vi "Main Engine.vi"() -> ()   [LabVIEW 2014, in "Dragon Tamers.lvlib"]
uses:
  Dragon Tamers.lvlib
  Typedefs/Queue Commands.ctl
  Typedefs/Main Cluster.ctl
  Typedefs/Config File Cluster.ctl
  Typedefs/Paths.ctl
  Typedefs/Input Parsed.ctl
  Typedefs/King.ctl
  Typedefs/Cell Pos.ctl
  Typedefs/Board.ctl
  Typedefs/Board Cell.ctl
  Typedefs/Cell Occupancy.ctl
  <vilib>/Utility/config.llb/NI_LVConfig.lvlib
  <vilib>/Utility/error.llb/DialogType.ctl
panel:
  out "Debug Board 2D String":string[][](table)
  out "Output Text":string
  out "Total Plays":i32=1
  out "Our Team":i32
  in  "Continue?":bool
  in  "Next Button":bool
  in  "Play Number":i32=1
  in  "Debug?":bool
  in  "Stop Waiting":bool
  out "Status":string
  in  "Stop Button":bool
  # "Dragon Tamers!"
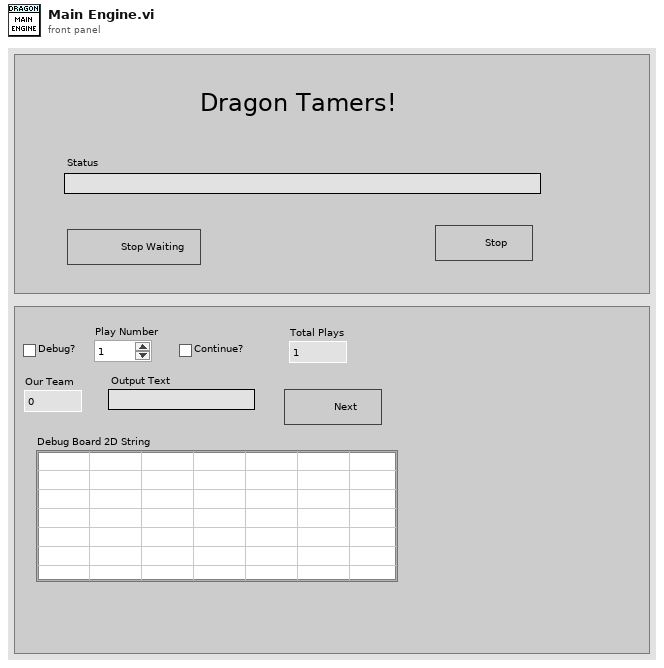
[diagram p1: front panel]
types:
  T1 = typedef "Dragon Tamers.lvlib/Queue Commands.ctl" = enum16{"Create", "Enqueue", "Enqueue N", "Enstack", "Dequeue", "Flush", "Release"}
  T2 = typedef "Dragon Tamers.lvlib/Main Cluster.ctl" = cluster{string, "Config":T3, "Paths":T4, "Play Number":i32, "Input Parsed":T5, "Output Text":string, "File List to Monitor":string[]}
  T3 = typedef "Dragon Tamers.lvlib/Config File Cluster.ctl" = cluster{"File Directory":path}
  T4 = typedef "Dragon Tamers.lvlib/Paths.ctl" = cluster{"App Directory":path, "Config File":path}
  T5 = typedef "Dragon Tamers.lvlib/Input Parsed.ctl" = cluster{"Our Team":i32, "King":T6, "Board":T8, "1D Board":T9[]}
  T6 = typedef "Dragon Tamers.lvlib/King.ctl" = cluster{"Set King?":bool, "Min":i32, "Max":i32, "DT Swap Count":i32, "Opp. Swap Count":i32, "DT Pos.":T7, "Opp. Pos.":T7}
  T7 = typedef "Dragon Tamers.lvlib/Cell Pos.ctl" = cluster{"X":i32, "Y":i32}
  T8 = typedef "Dragon Tamers.lvlib/Board.ctl" = T9[][]
  T9 = typedef "Dragon Tamers.lvlib/Board Cell.ctl" = cluster{"Team":i32, "Occu.":T10, "Count":i32}
  T10 = typedef "Dragon Tamers.lvlib/Cell Occupancy.ctl" = enum16{"N", "C", "K"}
  T11 = typedef "Dragon Tamers.lvlib/Parsed Board.ctl" = cluster{"DT King":i32, "Opp King":i32, "Count":i32[], "Empty Cells":i32[], "DT Cells":i32[], "Opp Cells":i32[], "DT Team":i32, "Opp. Team":i32}
  T12 = typedef "NI_LVConfig.lvlib/Config Data RefNum.ctl" = refnum<k1>
  T13 = typedef "DialogType.ctl" = u16
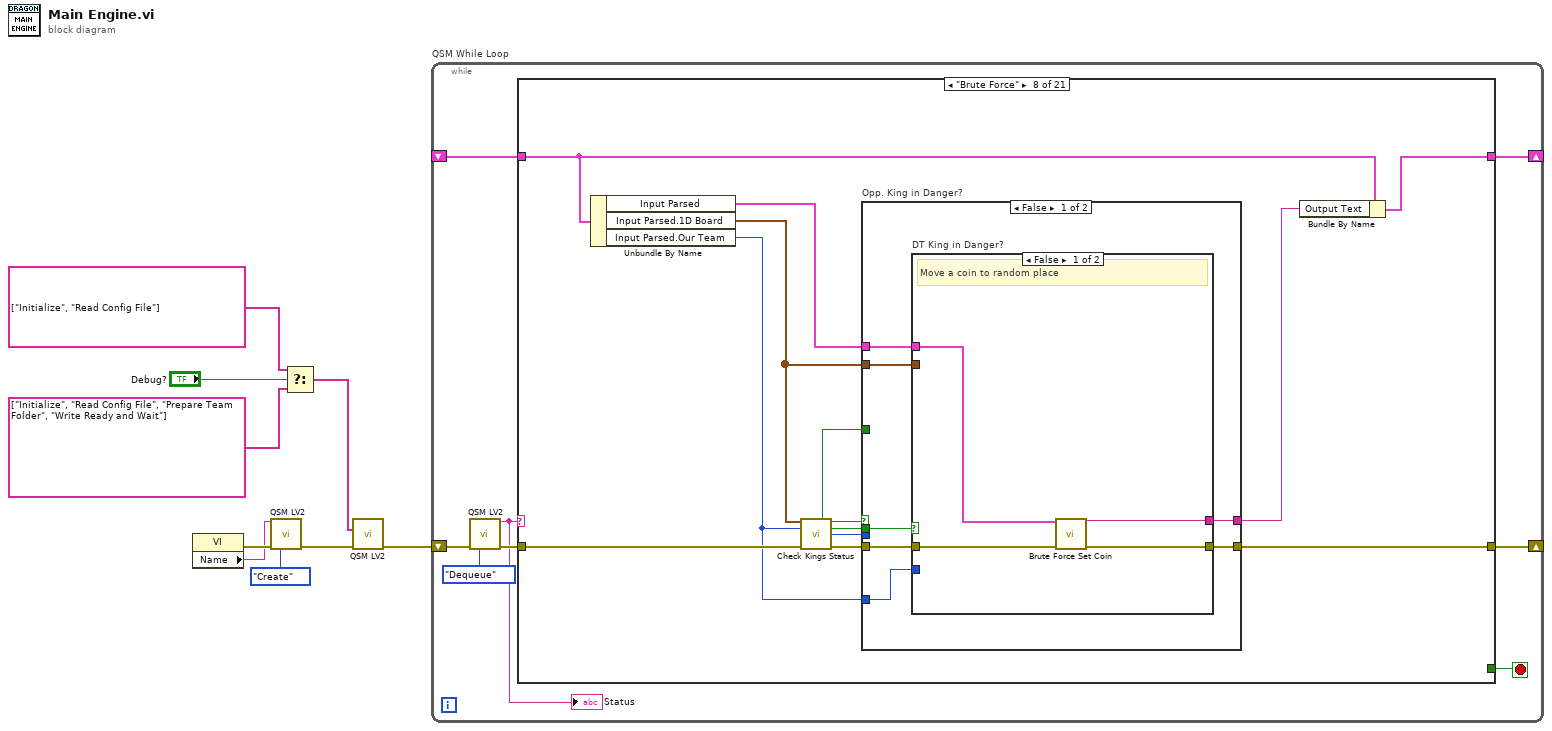
[diagram p0: block diagram]
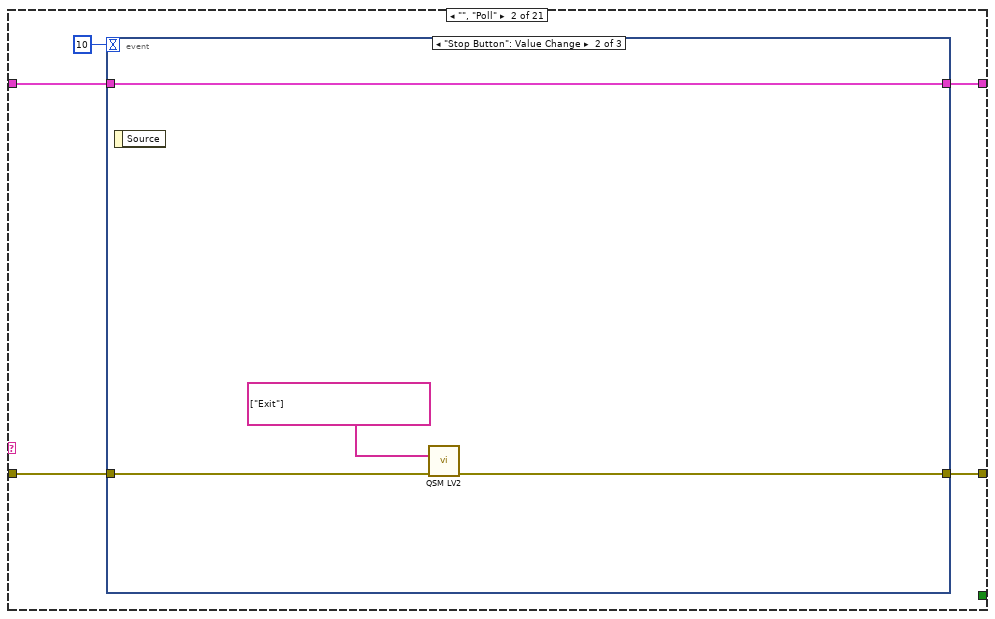
[diagram p3: hidden frame]
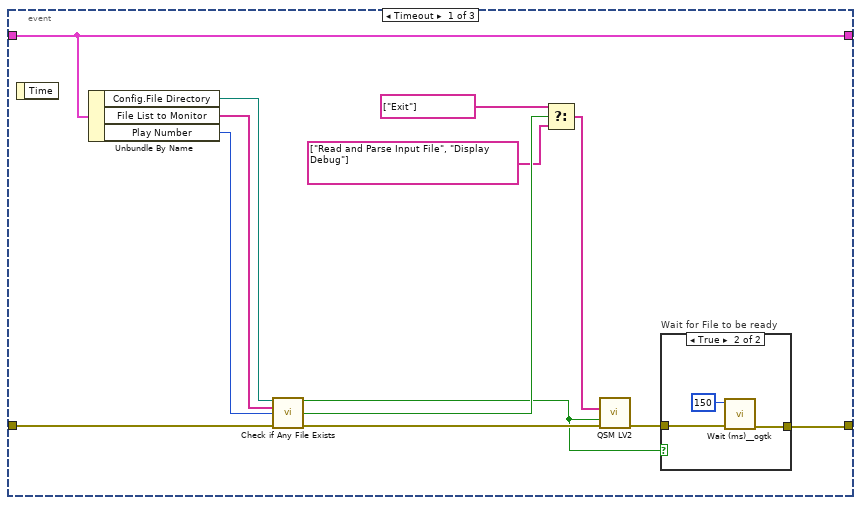
[diagram p4: hidden frame]
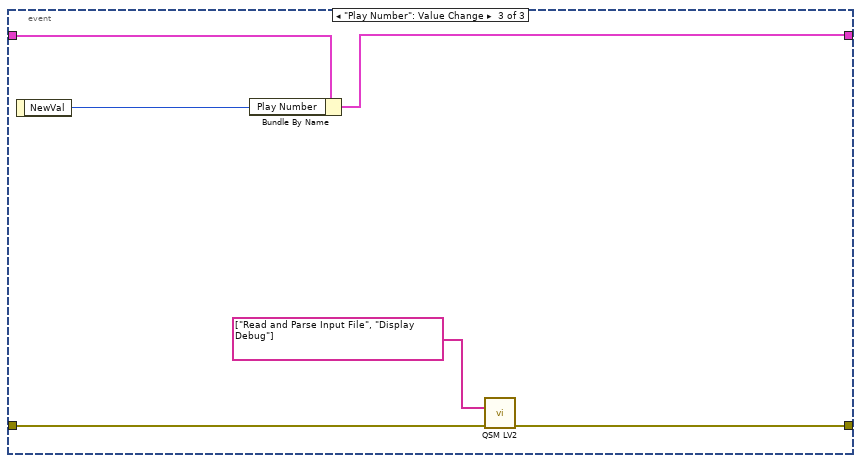
[diagram p6: hidden frame]
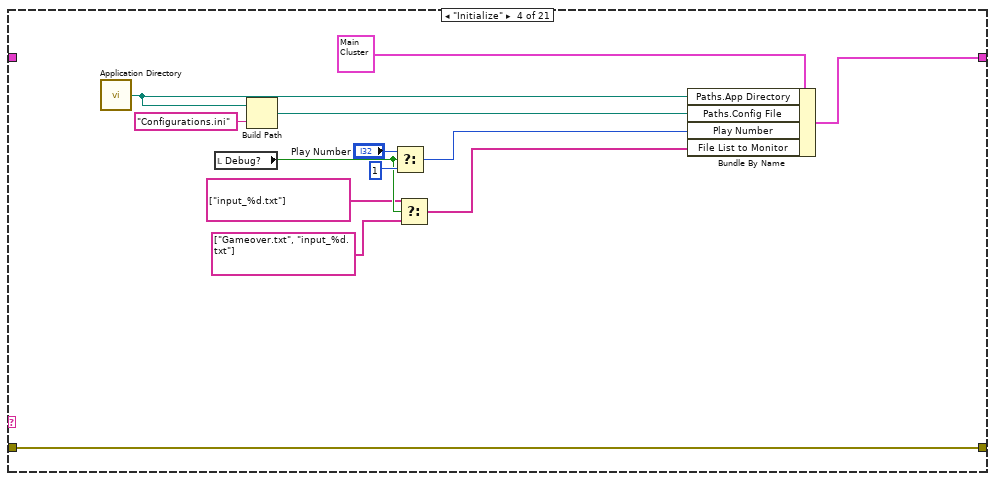
[diagram p8: hidden frame]
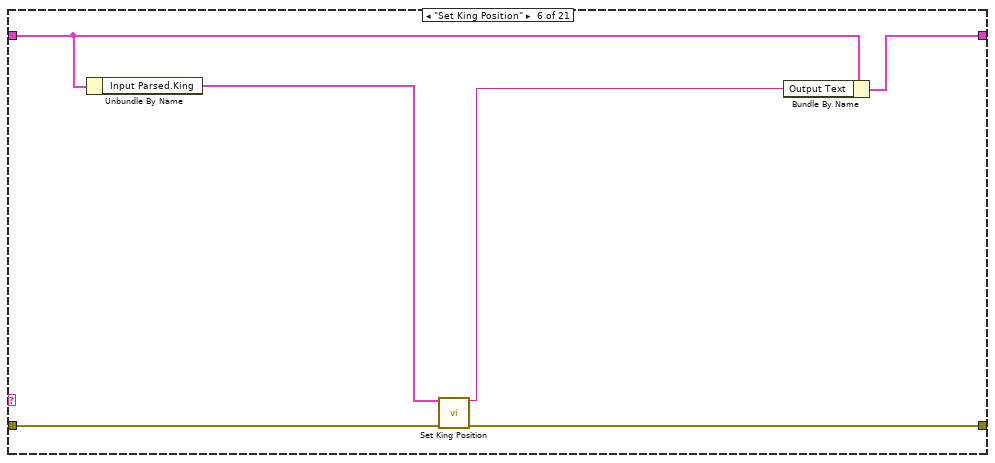
[diagram p10: hidden frame]
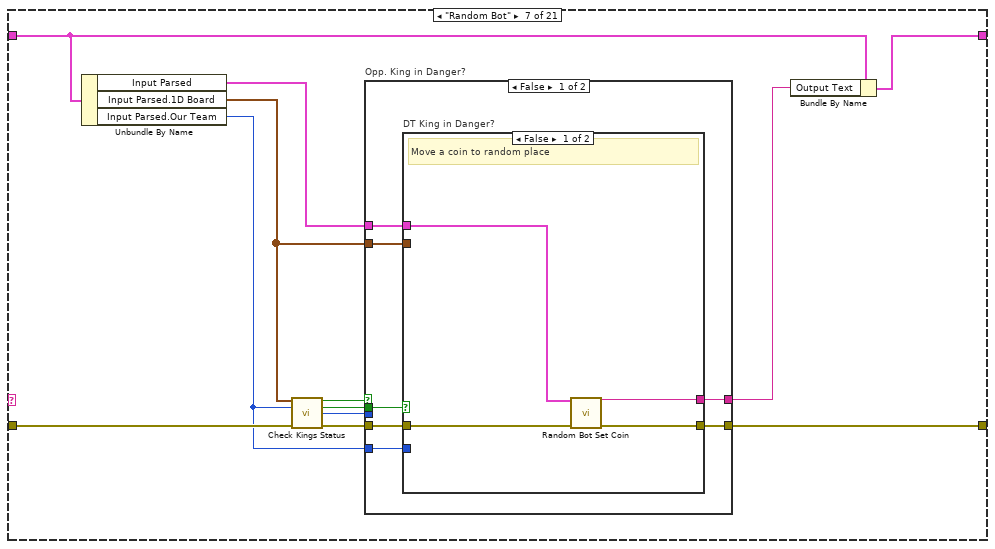
[diagram p11: hidden frame]
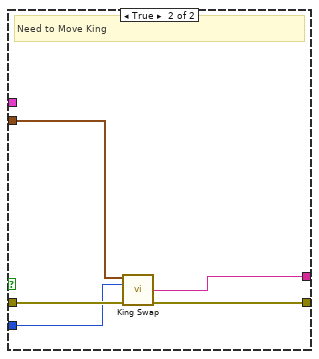
[diagram p12: hidden frame]
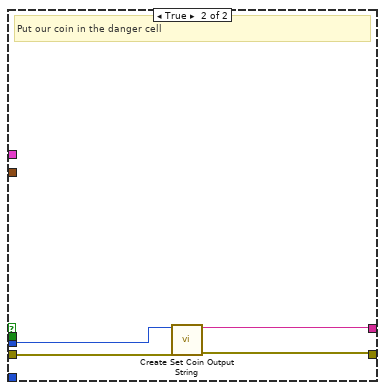
[diagram p13: hidden frame]
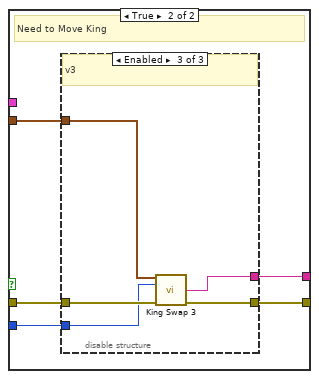
[diagram p14: hidden frame]
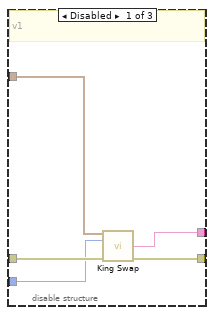
[diagram p15: hidden frame]
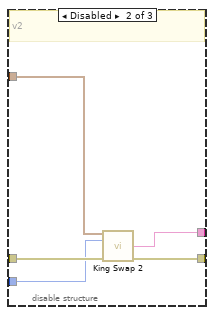
[diagram p16: hidden frame]
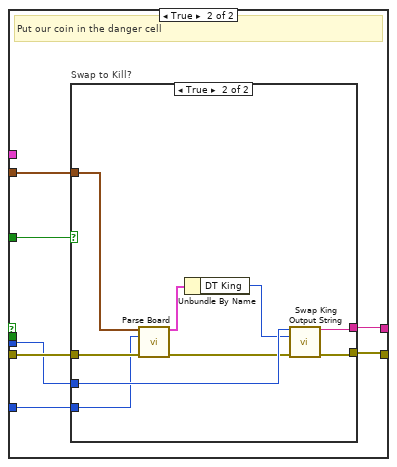
[diagram p17: hidden frame]
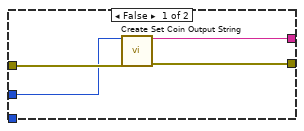
[diagram p18: hidden frame]
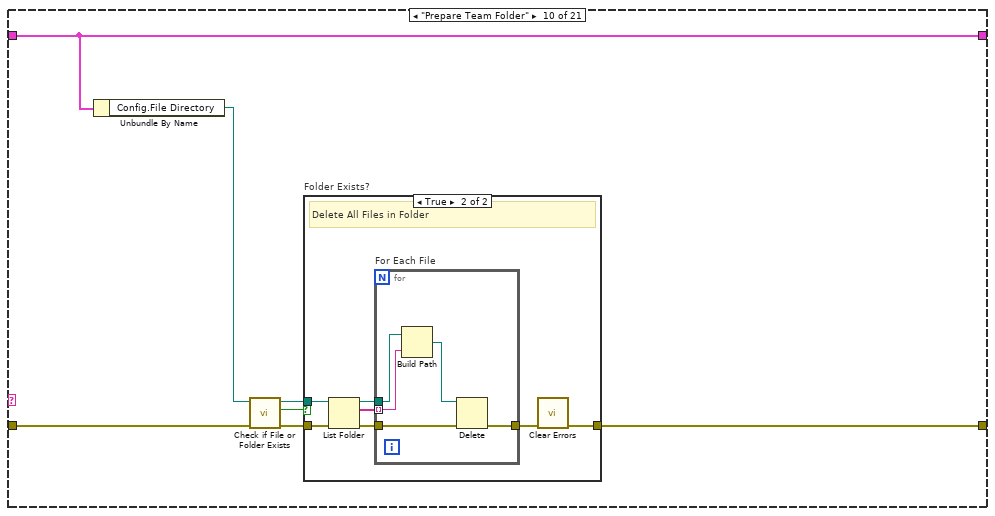
[diagram p20: hidden frame]
diagram:
  n1 = property class="VI"() -> (error out=w9:errorcluster, "Name"=w8:string)  [unwired: 2 in, 1 out]
  n2 = call "QSM LV2.vi"("Queue Name"=w8, "Error In"=w9, "Command"=Queue_Commands."Create") -> ("Error Out"=w6:errorcluster)  [unwired: 11 in, 1 out]
  n3 = Select(t=string[] ["Initialize", "Read Config File"] ("Enqueue N"), s="Debug?", f=string[] ["Initialize", "Read Config File", "Prepare Team Folder", "Write Ready and Wait"] ("Enqueue N")) -> (s? t:f=w4:string[])
  n4 = call "QSM LV2.vi"("Enqueue N"=w4, "Error In"=w6) -> ("Error Out"=w5:errorcluster)  [unwired: 12 in, 1 out]
  n5 = while "QSM While Loop" {
    shift-right: [w14] -> _
    shift-left: w5 -> [w17]
    shift-right: [w12] -> _
    shift-left: _ -> [w11]
    stop <- w13 stop-if-true
    n6 = call "QSM LV2.vi"("Error In"=w17, "Command"=Queue_Commands."Dequeue") -> ("Dequeue"=w10:string, "Error Out"=w15:errorcluster)  [unwired: 12 in]
    "Status" <- w10
    n7 = case "QSM Case Structure" shown="\"Brute Force\"" w10 {
      selector: w10 -> [_ _ _ _ _ _ _ _ _ _ _ _ _ _ _ _ _ _ _ w288 _]
      tunnel: w15 -> [w19 w22 w53 w66 w68 w74 w81 w114 w172 w177 w207 w214 w235 w249 w251 w261 w276 w280 w286 w291 w294]
      tunnel: [w19 w23 w53 w66 w68 w73 w84 w117 w172 w173 w204 w210 w231 w237 w251 w256 w276 w277 w286 w291 w293] -> w14
      tunnel: [_ _ _ _ _ _ _ _ _ _ _ _ _ _ _ _ _ _ _ _ TRUE] -> w13
      tunnel: [w18 w20 w52 w64 w67 w70 w85 w118 w171 w179 w197 w213 w233 w241 w250 w264 w275 w279 w285 w290 w292] -> w12
      tunnel: w11 -> [w18 w21 w52 _ w67 w71 w86 w119 w171 w179 w198 w213 w234 w242 w250 w264 w275 w279 w285 w290 w292]
      frame "/**** Poll ****/" {
      }
      frame "", "Poll" {
        n8 = event shown="[1] \"Stop Button\": Value Change" {
          selector: _ -> [_ _ _]
          dyn-events: _ -> [_ _ _]
          timeout: 10 -> [_ _ _]
          tunnel: [w26 w43 w47] -> w23
          tunnel: w22 -> [w37 w44 w48]
          tunnel: w21 -> [w36 w45 w51]
          tunnel: [w36 w45 w50] -> w20
          event Timeout {
            n9 = event-data() -> ()  [unwired: 1 in, 1 out]
            n10 = Unbundle By Name(w36) -> ("Config.File Directory"=w35:path, "File List to Monitor"=w25:string[], "Play Number"=w34:i32)
            n11 = call "Check if Any File Exists.vi"("File Directory"=w35, "File Names"=w25, "Play Number"=w34, "error in (no error)"=w37) -> ("File Found?"=w27:bool, "Game Over?"=w32:bool, "error out"=w33:errorcluster)  [unwired: 8 in, 1 out]
            n12 = Select(t=string[] ["Exit"], s=w32, f=string[] ["Read and Parse Input File", "Display Debug"]) -> (s? t:f=w29:string[])
            n13 = call "QSM LV2.vi"("Enqueue N"=w29, "Enqueue? (T)"=w27, "Error In"=w33) -> ("Error Out"=w28:errorcluster)  [unwired: 11 in, 1 out]
            n14 = case "Wait for File to be ready" shown="True" w27 {
              tunnel: w28 -> [w38 w41]
              tunnel: [w38 w40] -> w26
              frame False {
              }
              frame True {
                n15 = call <userlib>:"Wait (ms)__ogtk.vi"("error in (no error)"=w41, "milliseconds to wait"=u32 150) -> ("error out"=w40:errorcluster)  [unwired: 8 in, 1 out]
              }
            }
          }
          event "Stop Button": Value Change {
            n16 = event-data() -> ()  [unwired: 1 in, 1 out]
            n17 = call "QSM LV2.vi"("Enqueue N"=string[] ["Exit"], "Error In"=w44) -> ("Error Out"=w43:errorcluster)  [unwired: 12 in, 1 out]
          }
          event "Play Number": Value Change {
            n18 = event-data() -> ("NewVal"=w49:i32)  [unwired: 1 in]
            n19 = Bundle By Name(cluster=w51, "Play Number"=w49) -> (w50:T2)
            n20 = call "QSM LV2.vi"("Enqueue N"=string[] ["Read and Parse Input File", "Display Debug"], "Error In"=w48) -> ("Error Out"=w47:errorcluster)  [unwired: 12 in, 1 out]
          }
        }
      }
      frame "/**** Initialize ****/" {
      }
      frame "Initialize" {
        n21 = call <vilib>:"Application Directory.vi"() -> ("Application Directory"=w63:path)
        n22 = local read "Debug?"() -> (w56:bool)
        n23 = Build Path(base path=w63, name or relative path="Configurations.ini") -> (appended path=w61:path)
        n24 = Select(t="Play Number", s=w56, f=1 ("Play Number")) -> (s? t:f=w60:i32)
        n25 = Select(t=string[] ["input_%d.txt"] ("File Names"), s=w56, f=string[] ["Gameover.txt", "input_%d.txt"] ("File Names")) -> (s? t:f=w54:string[])
        n26 = Bundle By Name(cluster=T2 {"", "Config"={"File Directory"=path ""}, "Paths"={"App Directory"=path "", "Config File"=path ""}, "Play Number"=0, "Input Parsed"={"Our Team"=0, "King"={"Set King?"=FALSE, "Min"=0, "Max"=0, "DT Swap Count"=0, "Opp. Swap Count"=0, "DT Pos."={"X"=0, "Y"=0}, "Opp. Pos."={"X"=0, "Y"=0}}, "Board"=[], "1D Board"=[]}, "Output Text"="", "File List to Monitor"=["Gameover.txt", "input_%d.txt"]}, "Paths.App Directory"=w63, "Paths.Config File"=w61, "Play Number"=w60, "File List to Monitor"=w54) -> (w64:T2)
      }
      frame "/*** Algorithm ***/" {
      }
      frame "Set King Position" {
        n27 = Unbundle By Name(w71) -> ("Input Parsed.King"=w72:T6)
        n28 = call "Set King Position.vi"("King"=w72, "error in (no error)"=w74) -> ("King Set Output"=w69:string, "error out"=w73:errorcluster)  [unwired: 12 in]
        n29 = Bundle By Name(cluster=w71, "Output Text"=w69) -> (w70:T2)
      }
      frame "Random Bot" {
        n30 = Unbundle By Name(w86) -> ("Input Parsed"=w83:T5, "Input Parsed.1D Board"=w76:T9[], "Input Parsed.Our Team"=w75:i32)
        n31 = call "Check Kings Status.vi"("1D Board"=w76, "DT Team"=w75, "error in (no error)"=w81) -> ("Opp. King in Danger?"=w79:bool, "DT King in Danger?"=w77:bool, "Opp. King Danger Cell"=w78:i32, "error out"=w80:errorcluster)  [unwired: 7 in, 2 out]
        n32 = case "Opp. King in Danger?" shown="False" w79 {
          tunnel: [w93 w105] -> w84
          tunnel: w83 -> [w92 _]
          tunnel: [w91 w103] -> w82
          tunnel: w80 -> [w90 w106]
          tunnel: w78 -> [_ w104]
          tunnel: w77 -> [w89 _]
          tunnel: w76 -> [w88 _]
          tunnel: w75 -> [w87 _]
          frame False {
            n33 = case "DT King in Danger?" shown="False" w89 {
              tunnel: [w97 w101] -> w93
              tunnel: w92 -> [w96 _]
              tunnel: [w95 w98] -> w91
              tunnel: w90 -> [w94 w102]
              tunnel: w88 -> [_ w100]
              tunnel: w87 -> [_ w99]
              frame False {
                # "Move a coin to random place"
                n34 = call "Random Bot Set Coin.vi"("Input Parsed"=w96, "error in (no error)"=w94) -> ("Output Text"=w95:string, "error out"=w97:errorcluster)  [unwired: 12 in]
              }
              frame True {
                # "Need to Move King"
                n35 = call "King Swap.vi"("1D Board"=w100, "DT Team #"=w99, "error in (no error)"=w102) -> ("Output Text"=w98:string, "error out"=w101:errorcluster)  [unwired: 9 in, 2 out]
              }
            }
          }
          frame True {
            # "Put our coin in the danger cell"
            n36 = call "Create Set Coin Output String.vi"("Cell Index"=w104, "error in (no error)"=w106) -> ("Output Text"=w103:string, "error out"=w105:errorcluster)  [unwired: 12 in]
          }
        }
        n37 = Bundle By Name(cluster=w86, "Output Text"=w82) -> (w85:T2)
      }
      frame "Brute Force" {
        n38 = Unbundle By Name(w119) -> ("Input Parsed"=w116:T5, "Input Parsed.1D Board"=w109:T9[], "Input Parsed.Our Team"=w108:i32)
        n39 = call "Check Kings Status.vi"("1D Board"=w109, "DT Team"=w108, "error in (no error)"=w114) -> ("Swap to Kill Opp. King?"=w107:bool, "Opp. King in Danger?"=w112:bool, "DT King in Danger?"=w110:bool, "Opp. King Danger Cell"=w111:i32, "error out"=w113:errorcluster)  [unwired: 7 in, 1 out]
        n40 = case "Opp. King in Danger?" shown="False" w112 {
          tunnel: [w126 w156] -> w117
          tunnel: w116 -> [w125 _]
          tunnel: [w124 w154] -> w115
          tunnel: w113 -> [w123 w157]
          tunnel: w111 -> [_ w155]
          tunnel: w110 -> [w122 _]
          tunnel: w109 -> [w121 w152]
          tunnel: w108 -> [w120 w151]
          tunnel: w107 -> [_ w153]
          frame False {
            n41 = case "DT King in Danger?" shown="False" w122 {
              tunnel: [w130 w134] -> w126
              tunnel: w125 -> [w129 _]
              tunnel: [w128 w131] -> w124
              tunnel: w123 -> [w127 w135]
              tunnel: w121 -> [_ w133]
              tunnel: w120 -> [_ w132]
              frame False {
                # "Move a coin to random place"
                n42 = call "Brute Force Set Coin.vi"("Input Parsed"=w129, "error in (no error)"=w127) -> ("Output Text"=w128:string, "error out"=w130:errorcluster)  [unwired: 12 in]
              }
              frame True {
                # "Need to Move King"
                n43 = disable-structure shown="Enabled" {
                  disable-tunnel: w135 -> [w140 w145 w150]
                  disable-tunnel: [w139 w144 w149] -> w134
                  disable-tunnel: w133 -> [w138 w143 w148]
                  disable-tunnel: w132 -> [w137 w142 w147]
                  disable-tunnel: [w136 w141 w146] -> w131
                  frame Disabled {
                    # "v1"
                    n44 = call "King Swap.vi"("1D Board"=w138, "DT Team #"=w137, "error in (no error)"=w140) -> ("Output Text"=w136:string, "error out"=w139:errorcluster)  [unwired: 9 in, 2 out]
                  }
                  frame Disabled {
                    # "v2"
                    n45 = call "King Swap 2.vi"("1D Board"=w143, "DT Team #"=w142, "error in (no error)"=w145) -> ("Output Text"=w141:string, "error out"=w144:errorcluster)  [unwired: 9 in, 2 out]
                  }
                  frame Enabled {
                    # "v3"
                    n46 = call "King Swap 3.vi"("1D Board"=w148, "DT Team #"=w147, "error in (no error)"=w150) -> ("Output Text"=w146:string, "error out"=w149:errorcluster)  [unwired: 9 in, 2 out]
                  }
                }
              }
            }
          }
          frame True {
            # "Put our coin in the danger cell"
            n47 = case "Swap to Kill?" shown="True" w153 {
              tunnel: w157 -> [w161 w167]
              tunnel: [w160 w170] -> w156
              tunnel: w155 -> [w159 w168]
              tunnel: [w158 w169] -> w154
              tunnel: w152 -> [_ w165]
              tunnel: w151 -> [_ w163]
              frame False {
                n48 = call "Create Set Coin Output String.vi"("Cell Index"=w159, "error in (no error)"=w161) -> ("Output Text"=w158:string, "error out"=w160:errorcluster)  [unwired: 12 in]
              }
              frame True {
                n49 = call "Parse Board.vi"("Board Array"=w165, "DT Team #"=w163, "error in (no error)"=w167) -> ("Parsed Board Info"=w164:T11, "error out"=w166:errorcluster)  [unwired: 11 in]
                n50 = Unbundle By Name(w164) -> ("DT King"=w162:i32)
                n51 = call "Swap King Output String.vi"("New Cell Index"=w168, "Old Cell Index"=w162, "error in (no error)"=w166) -> ("Output Text"=w169:string, "error out"=w170:errorcluster)  [unwired: 11 in]
              }
            }
          }
        }
        n52 = Bundle By Name(cluster=w119, "Output Text"=w115) -> (w118:T2)
      }
      frame "/*** File Handling ***/" {
      }
      frame "Prepare Team Folder" {
        n53 = Unbundle By Name(w179) -> ("Config.File Directory"=w178:path)
        n54 = call <vilib>:"Check if File or Folder Exists.vi"("error in (no error)"=w177, "path"=w178) -> ("error out"=w174:errorcluster, "file or folder exists?"=w176:bool, "dup path"=w175:path)  [unwired: 7 in]
        n55 = case "Folder Exists?" shown="True" w176 {
          tunnel: w175 -> [w180 w189]
          tunnel: w174 -> [w182 w188]
          tunnel: [w181 w183] -> w173
          frame False {
            # "Create Folder"
            n56 = Create Folder(path (use dialog)=w180, error in=w182) -> (error out=w181:errorcluster)  [unwired: 1 in, 2 out]
          }
          frame True {
            # "Delete All Files in Folder"
            n57 = List Folder(path=w189, error in=w188) -> (path out=w187:path, filenames=w186:string[], error out=w185:errorcluster)  [unwired: 2 in, 1 out]
            n58 = for "For Each File" {
              tunnel: w187 -> [w194]
              tunnel: w186 -> [w193] mode=indexing
              tunnel: w185 -> [w191]
              tunnel: [w190] -> w184
              n59 = Build Path(base path=w194, name or relative path=w193) -> (appended path=w192:path)
              n60 = Delete(path (use dialog)=w192, error in=w191) -> (error out=w190:errorcluster)  [unwired: 3 in, 2 out]
            }
            n61 = call <vilib>:"Clear Errors.vi"("error in (no error)"=w184) -> ("error out"=w183:errorcluster)  [unwired: 5 in, 1 out]
          }
        }
      }
      frame "Read Config File" {
        n62 = Unbundle By Name(w198) -> ("Config"=w199:T3, "Paths.Config File"=w203:path)
        n63 = call <vilib>:"Open Config Data.vi"("error in (no error)"=w207, "configuration file path"=w203) -> ("error out"=w206:errorcluster, "refnum"=w202:T12)  [unwired: 7 in, 1 out]
        n64 = call <userlib>:"Read INI Cluster__ogtk.vi"("error in (no error)"=w206, "INI Fomatted Cluster Type"=w199, "refnum"=w202) -> ("error out"=w205:errorcluster, "INI Fomatted Cluster"=w200:variant, "dup refnum"=w195:T12)  [unwired: 4 in, 2 out]
        n65 = Variant To Data(error in=w205, type=w199, Variant=w200) -> (data=w196:T3, error out=w201:errorcluster)
        n66 = call <vilib>:"Close Config Data.vi"("error in (no error)"=w201, "refnum"=w195) -> ("error out"=w204:errorcluster)  [unwired: 8 in, 1 out]
        n67 = Bundle By Name(cluster=w198, "Config"=w196) -> (w197:T2)
      }
      frame "Write Ready and Wait" {
        n68 = Unbundle By Name(w213) -> ("Config.File Directory"=w212:path)
        n69 = while "Wait till input_1.txt is created" {
          tunnel: w212 -> [w218]
          tunnel: w214 -> [w219]
          tunnel: [w216] -> w211
          tunnel: [w217] -> w209
          stop <- w220 stop-if-true
          n70 = Wait (ms)(milliseconds to wait=u32 100) -> ()  [unwired: 1 out]
          n71 = call "Write Ready and Wait.vi"("File Directory"=w218, "error in (no error)"=w219) -> ("Stop?"=w215:bool, "Exit?"=w217:bool, "error out"=w216:errorcluster)  [unwired: 11 in]
          n72 = Compound Arithmetic op=OR(w215, "Stop Waiting") -> (w220:bool)
        }
        n73 = call "QSM LV2.vi"("Enqueue N"=string[] ["Exit"], "Enqueue? (T)"=w209, "Error In"=w211) -> ("Error Out"=w210:errorcluster)  [unwired: 11 in, 1 out]
      }
      frame "Read and Parse Input File" {
        n74 = Unbundle By Name(w234) -> ("Input Parsed"=w223:T5, "Config.File Directory"=w224:path, "Play Number"=w225:i32)
        n75 = call "Read and Parse Input File.vi"("Input Parsed"=w223, "Directory Path"=w224, "Play Number"=w225, "error in (no error)"=w235) -> ("Input Parsed"=w230:T5, "error out"=w232:errorcluster)  [unwired: 10 in]
        n76 = Unbundle By Name(w230) -> ("King.Set King?"=w229:bool)
        n77 = Select(t=string[] ["Set King Position", "Write Output"], s=w229, f=string[] ["Brute Force", "Write Output"]) -> (s? t:f=w226:string[])
        n78 = Bundle By Name(cluster=w234, "Input Parsed"=w230) -> (w233:T2)
        n79 = call "QSM LV2.vi"("Enqueue N"=w226, "Error In"=w232) -> ("Error Out"=w231:errorcluster)  [unwired: 12 in, 1 out]
      }
      frame "Write Output" {
        n80 = Unbundle By Name(w242) -> ("Play Number"=w239:i32, "Config.File Directory"=w246:path, "Output Text"=w243:string)
        "Output Text" <- w243
        n81 = Format Into String(format string="output_%d.txt", error in=w249, w239) -> (resulting string=w245:string, error out=w248:errorcluster)  [unwired: 1 in]
        n82 = Build Path(base path=w246, name or relative path=w245) -> (appended path=w244:path)
        n83 = Write to Text File(file (use dialog)=w244, text=w243, error in=w248) -> (error out=w238:errorcluster)  [unwired: 1 in, 2 out]
        n84 = Increment(x=w239) -> (x+1=w240:i32)
        n85 = call <userlib>:"Wait (ms)__ogtk.vi"("error in (no error)"=w238, "milliseconds to wait"=u32 200) -> ("error out"=w237:errorcluster)  [unwired: 8 in, 1 out]
        n86 = Bundle By Name(cluster=w242, "Play Number"=w240) -> (w241:T2)
      }
      frame "/*** Debug ***/" {
      }
      frame "Display Debug" {
        n87 = Unbundle By Name(w264) -> ("Input Parsed.Our Team"=→"Our Team":i32, "Input Parsed.1D Board"=w253:T9[], "Play Number"=w258:i32, "Config.File Directory"=w260:path)
        n88 = call "Get Total Plays.vi"("File Directory"=w260, "error in (no error)"=w261) -> ("Total Plays"=→"Total Plays":i32, "error out"=w257:errorcluster)  [unwired: 12 in]
        n89 = local write "Play Number"(w258) -> ()
        n90 = local read "Debug?"() -> (w263:bool)
        n91 = control-ref of="Debug Board 2D String"() -> (w252:refnum<vi>)
        n92 = case shown="True" w263 {
          tunnel: w258 -> [_ w266]
          tunnel: [_ w265] -> w255
          frame False {
          }
          frame True {
            n93 = while {
              tunnel: w266 -> [w269]
              tunnel: ["Stop Button"] -> w265
              stop <- w271 stop-if-true
              n94 = local read "Play Number"() -> (w270:i32)
              n95 = Not Equal?(x=w270, y=w269) -> (x != y?=w268:bool)
              n96 = Wait (ms)(milliseconds to wait=u32 100) -> ()  [unwired: 1 out]
              n97 = Compound Arithmetic op=OR(w268, "Continue?", "Next Button", "Stop Button") -> (w271:bool)
            }
          }
        }
        n98 = call "1D Cluster to Color Table.vi"("1D Board"=w253, "Debug Board 2D String Ref"=w252) -> ()  [unwired: 10 in]
        n99 = call "QSM LV2.vi"("Enqueue N"=string[] ["Exit"], "Enqueue? (T)"=w255, "Error In"=w257) -> ("Error Out"=w256:errorcluster)  [unwired: 11 in, 1 out]
      }
      frame "/*** Error Handler ***/" {
      }
      frame "Error" {
        n100 = disable-structure shown="Enabled" {
          disable-tunnel: w280 -> [w283 w284]
          disable-tunnel: [w282 w284] -> w278
          frame Disabled {
            w281 = T13 2 items=["no dialog", "OK message", "continue or stop message", "OK message + warnings", "continue/stop + warnings"] ("type of dialog (OK msg:1)")
            n101 = call <vilib>:"Simple Error Handler.vi"("type of dialog (OK msg:1)"=w281, "error in (no error)"=w283) -> ("error out"=w282:errorcluster)  [unwired: 3 in, 4 out]
          }
          frame Enabled {
          }
        }
        n102 = call <vilib>:"Clear Errors.vi"("error in (no error)"=w278) -> ("error out"=w277:errorcluster)  [unwired: 5 in, 1 out]
      }
      frame "/**** Exit ****/" {
      }
      frame Default {
        n103 = Concatenate Strings("Unknown case - " ("string"), w288) -> (w287:string)
        n104 = One Button Dialog(message=w287) -> ()  [unwired: 1 in, 1 out]
      }
      frame "Exit" {
        n105 = call "QSM LV2.vi"("Error In"=w294, "Command"=Queue_Commands."Flush") -> ("Error Out"=w295:errorcluster)  [unwired: 12 in, 1 out]
        n106 = call "QSM LV2.vi"("Error In"=w295, "Command"=Queue_Commands."Release") -> ("Error Out"=w293:errorcluster)  [unwired: 12 in, 1 out]
      }
    }
  }
